vi "FieldOrientedTransform.vi"(9 "Joystick Y":dbl format="%.4f", 11 "Joystick X":dbl format="%.4f") -> (1 "Robot Y":dbl format="%.4f", 3 "Robot X":dbl format="%.4f")   [LabVIEW 2023, in "TShirtWork-SwerveDrive_ACT_ts.lvlib"]
doc: "Transforms X and Y joystick axes based on the robot's current orientation, allowing a swerve robot to be controlled in the field-oriented reference frame. The code is primarily based on code included in the FRC WPI Library."
uses:
  TShirtWork-SwerveDrive_ACT_ts.lvlib
panel:
  in  "Compass Heading(0-1)":dbl format="%.4f"
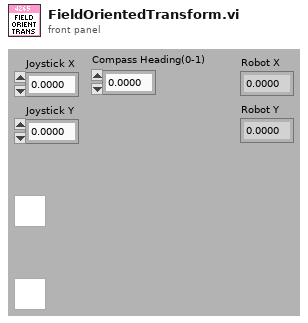
[diagram p1: front panel]
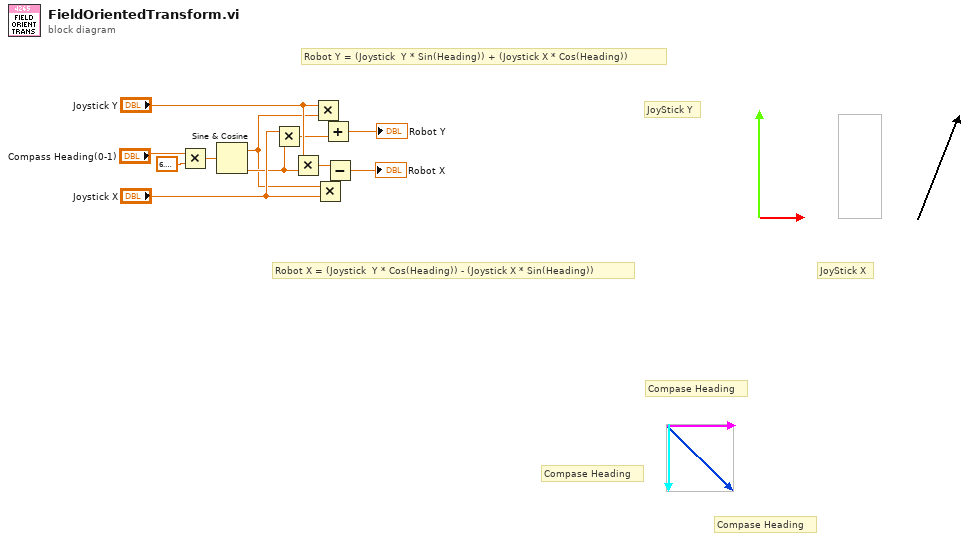
[diagram p0: block diagram]
diagram:
  # "Compase Heading"
  # "Compase Heading"
  # "Compase Heading"
  # "JoyStick X"
  # "JoyStick Y"
  # "Robot X = (Joystick  Y * Cos(Heading)) - (Joystick X * Sin(Heading))"
  # "Robot Y = (Joystick  Y * Sin(Heading)) + (Joystick X * Cos(Heading))"
  n1 = Multiply(x="Compass Heading(0-1)", y=6.283185307179586) -> (x*y=w3:dbl)
  n2 = Sine & Cosine(0:w3) -> (1:w1:dbl, 2:w2:dbl)
  n3 = Multiply(x="Joystick X", y=w2) -> (x*y=w5:dbl)
  n4 = Multiply(x="Joystick Y", y=w2) -> (x*y=w7:dbl)
  n5 = Multiply(x="Joystick Y", y=w1) -> (x*y=w6:dbl)
  n6 = Multiply(x=w1, y="Joystick X") -> (x*y=w8:dbl)
  n7 = Add(x=w6, y=w5) -> (x+y=→"Robot Y":dbl)
  n8 = Subtract(x=w7, y=w8) -> (x-y=→"Robot X":dbl)
